vi "refresh glyph set.vi"(8 "error in":errorcluster, 11 "glyph manager in":T1) -> (0 "error out":errorcluster, 3 "glyph manager out":T1)   [LabVIEW 2013, in "glyph manager.lvlib"]
uses:
  glyph manager.lvlib
  glyph manager.ctl
  <vilib>/picture/picture.llb/imagedata.ctl
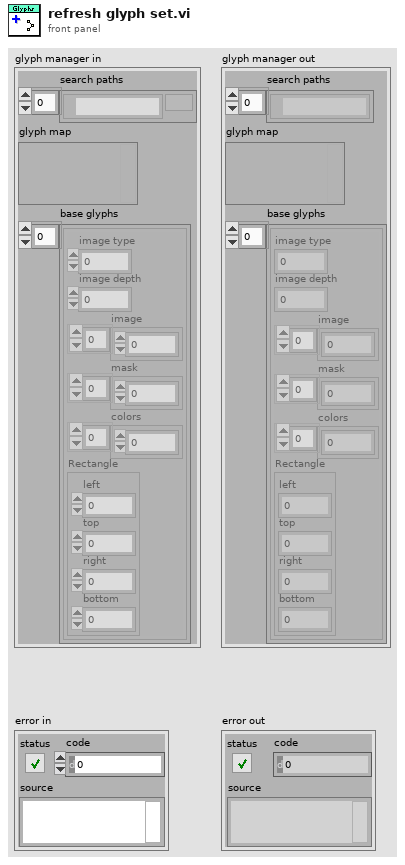
[diagram p1: front panel]
types:
  T1 = typedef "glyph manager.lvlib/glyph manager.ctl" = cluster{"search paths":path[], "glyph map":variant, "base glyphs":T2[]}
  T2 = typedef "imagedata.ctl" = cluster{"image type":i32, "image depth":i32, "image":u8[], "mask":u8[], "colors":u32[], "Rectangle":cluster{"left":i16, "top":i16, "right":i16, "bottom":i16}}
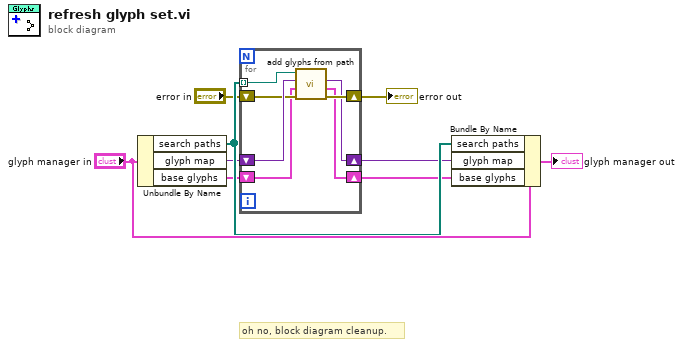
[diagram p0: block diagram]
diagram:
  # "oh no, block diagram cleanup."
  n1 = Unbundle By Name("glyph manager in") -> ("search paths"=w7:path[], "glyph map"=w6:variant, "base glyphs"=w5:T2[])
  n2 = for {
    tunnel: w7 -> [w16] mode=indexing
    shift-right: [w11] -> w4
    shift-left: w6 -> [w15]
    shift-right: [w10] -> w1
    shift-left: w5 -> [w12]
    shift-right: [w14] -> w2
    shift-left: "error in" -> [w13]
    n3 = call "add glyphs from path.vi"("error in (no error)"=w13, "base glyphs in"=w12, "glyph map in"=w15, "Path"=w16) -> ("error out"=w14:errorcluster, "base glyphs out"=w10:T2[], "glyph map out"=w11:variant)  [unwired: 5 in]
  }
  "error out" <- w2
  n4 = Bundle By Name(cluster="glyph manager in", "search paths"=w7, "glyph map"=w4, "base glyphs"=w1) -> (→"glyph manager out":T1)
